vi "Read Observer Directory.vi"(11 "ModuleConfigs in":refnum<class "ModuleConfigs.lvclass">) -> (2 "Observer Directory":string, 3 "ModuleConfigs out":refnum<class "ModuleConfigs.lvclass">)   [LabVIEW 2014, in "ModuleConfigs.lvclass"]
uses:
  ModuleConfigs.lvclass
  ModuleConfigs.lvclass/ModuleConfigs.ctl
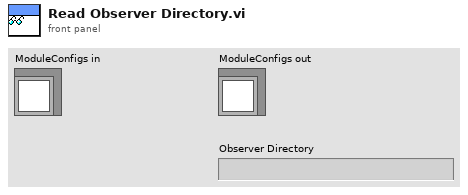
[diagram p1: front panel]
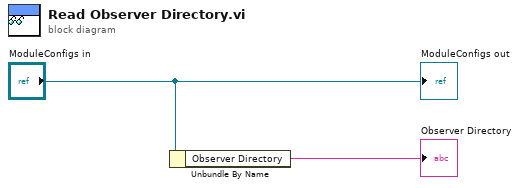
[diagram p0: block diagram]
diagram:
  n1 = Unbundle By Name("ModuleConfigs in") -> ("Observer Directory"=→"Observer Directory":string)
  "ModuleConfigs out" <- "ModuleConfigs in"
